vi "Drive Config.vi"(8 "error in (no error)":errorcluster, 11 "Config in":refnum<class "Config.lvclass">) -> (0 "error out":errorcluster, 1 "IDs found?":bool, 2 "Robot Drivetrain Data":T1={"Right"={"Talon"=0, "Victor1"=0, "Victor2"=0}, "Left"={"Talon"=0, "Victor1"=0, "Victor2"=0}, "Drive Velocity Low Gear"={"P"=0.0, "I"=0.0, "D"=0.0, "F"=0.0, "integralZone"=0.0, "allowableClosedLoopError"=0, "maxIntegralAccumulator"=0.0, "closedLoopPeakOutput"=1.0, "closedLoopPeriod"=1}, "Drive Velocity High Gear"={"P"=0.0, "I"=0.0, "D"=0.0, "F"=0.0, "integralZone"=0.0, "allowableClosedLoopError"=0, "maxIntegralAccumulator"=0.0, "closedLoopPeakOutput"=1.0, "closedLoopPeriod"=1}, "Drive Motion Magic Primary Low Gear"={"P"=0.0, "I"=0.0, "D"=0.0, "F"=0.0, "integralZone"=0.0, "allowableClosedLoopError"=0, "maxIntegralAccumulator"=0.0, "closedLoopPeakOutput"=1.0, "closedLoopPeriod"=1}, "Drive Motion Magic Primary High Gear"={"P"=0.0, "I"=0.0, "D"=0.0, "F"=0.0, "integralZone"=0.0, "allowableClosedLoopError"=0, "maxIntegralAccumulator"=0.0, "closedLoopPeakOutput"=1.0, "closedLoopPeriod"=1}, "Drive Motion Magic Secondary Low Gear"={"P"=0.0, "I"=0.0, "D"=0.0, "F"=0.0, "integralZone"=0.0, "allowableClosedLoopError"=0, "maxIntegralAccumulator"=0.0, "closedLoopPeakOutput"=1.0, "closedLoopPeriod"=1}, "Drive Motion Magic Secondary High Gear"={"P"=0.0, "I"=0.0, "D"=0.0, "F"=0.0, "integralZone"=0.0, "allowableClosedLoopError"=0, "maxIntegralAccumulator"=0.0, "closedLoopPeakOutput"=1.0, "closedLoopPeriod"=1}, "Drive Right Invert"=FALSE, "Drive Right Sensor Phase"=FALSE, "Drive Left Invert"=FALSE, "Drive Left Sensor Phase"=FALSE, "Low Gear Max Velocity"=0, "High Gear Max Velocity"=0, "Motion Magic Low Gear Max Velocity"=0, "Motion Magic Low Gear Max Acceleration"=0, "Motion Magic High Gear Max Velocity"=0, "Motion Magic High Gear Max Acceleration"=0}, 3 "Config out":refnum<class "Config.lvclass">, 4 "PIDFs found":bool, 5 "File Found?":bool)   [LabVIEW 2018, in "Config.lvlib" / "Config.lvclass"]
doc: "Use this VI to configure the drive. It will return both if it found the slots, as well as the PIDF values."
uses:
  Config.lvclass
  Controls/Drivetrain Data.ctl
  Drive/Pod Drive/Pod.ctl
  <vilib>/Rock Robotics/WPI/ThirdParty/Phoenix-LabVIEW/Motor Controller/Controls/CTRE_Phoenix_MotorControl_SlotStructure.ctl
  Drive/Pod Drive/Pod Drive.lvclass
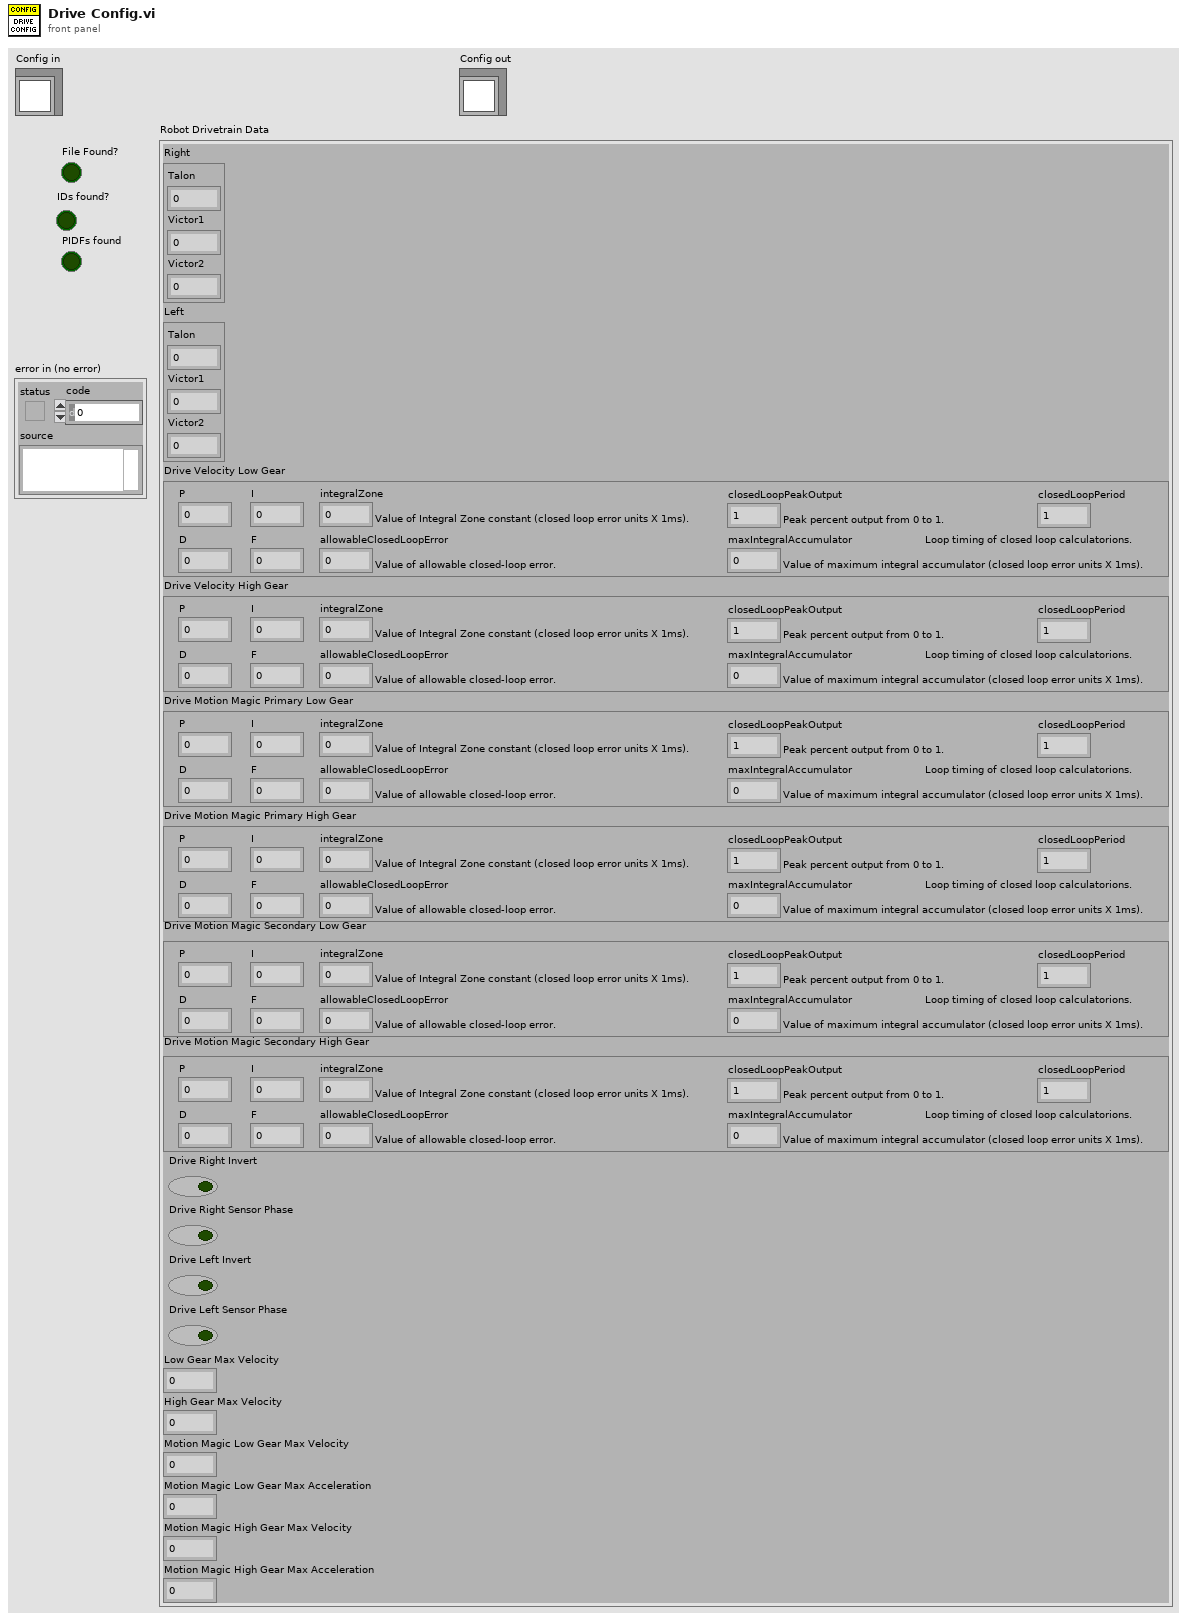
[diagram p1: front panel]
types:
  T1 = typedef "Config.lvlib/Config.lvclass/Drivetrain Data.ctl" = cluster{"Right":T2, "Left":T2, "Drive Velocity Low Gear":T3, "Drive Velocity High Gear":T3, "Drive Motion Magic Primary Low Gear":T3, "Drive Motion Magic Primary High Gear":T3, "Drive Motion Magic Secondary Low Gear":T3, "Drive Motion Magic Secondary High Gear":T3, "Drive Right Invert":bool, "Drive Right Sensor Phase":bool, "Drive Left Invert":bool, "Drive Left Sensor Phase":bool, "Low Gear Max Velocity":u32, "High Gear Max Velocity":u32, "Motion Magic Low Gear Max Velocity":u32, "Motion Magic Low Gear Max Acceleration":u32, "Motion Magic High Gear Max Velocity":u32, "Motion Magic High Gear Max Acceleration":u32}
  T2 = typedef "Drive.lvlib/Pod Drive.lvclass/Pod.ctl" = cluster{"Talon":u8, "Victor1":u8, "Victor2":u8}
  T3 = typedef "CTRE_Phoenix_MotorControl_SlotStructure.ctl" = cluster{"P":dbl, "I":dbl, "D":dbl, "F":dbl, "integralZone":dbl, "allowableClosedLoopError":i32, "maxIntegralAccumulator":dbl, "closedLoopPeakOutput":dbl, "closedLoopPeriod":i32}
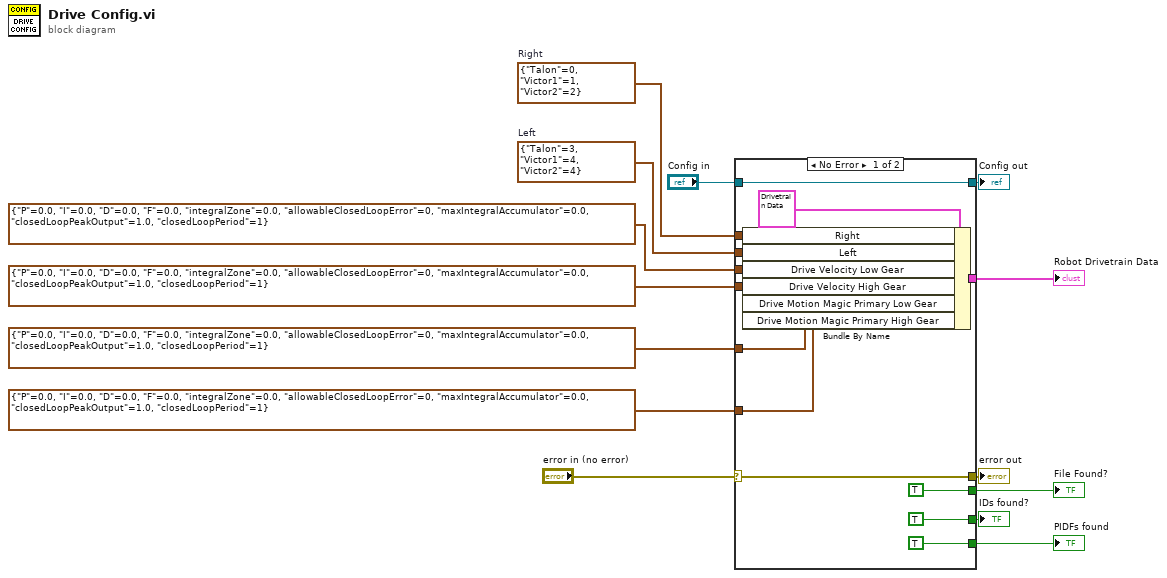
[diagram p0: block diagram]
diagram:
  w1 = T2 {"Talon"=3, "Victor1"=4, "Victor2"=4}  # Left
  w2 = T2 {"Talon"=0, "Victor1"=1, "Victor2"=2}  # Right
  n1 = case shown="No Error" "error in (no error)" {
    selector: "error in (no error)" -> [w26 w29]
    tunnel: [w26 w29] -> w13
    tunnel: [w27 w28] -> w11
    tunnel: "Config in" -> [w27 w28]
    tunnel: [TRUE ("File Found?") _] -> w10
    tunnel: [TRUE ("IDs found?") _] -> w9
    tunnel: [TRUE ("PIDFs found") _] -> w8
    tunnel: [w21 _] -> w7
    tunnel: T3 {"P"=0.0, "I"=0.0, "D"=0.0, "F"=0.0, "integralZone"=0.0, "allowableClosedLoopError"=0, "maxIntegralAccumulator"=0.0, "closedLoopPeakOutput"=1.0, "closedLoopPeriod"=1} ("PID Slot 0") -> [w20 _]
    tunnel: T3 {"P"=0.0, "I"=0.0, "D"=0.0, "F"=0.0, "integralZone"=0.0, "allowableClosedLoopError"=0, "maxIntegralAccumulator"=0.0, "closedLoopPeakOutput"=1.0, "closedLoopPeriod"=1} ("PID Slot 0") -> [w19 _]
    tunnel: T3 {"P"=0.0, "I"=0.0, "D"=0.0, "F"=0.0, "integralZone"=0.0, "allowableClosedLoopError"=0, "maxIntegralAccumulator"=0.0, "closedLoopPeakOutput"=1.0, "closedLoopPeriod"=1} ("PID Slot 0") -> [w18 _]
    tunnel: T3 {"P"=0.0, "I"=0.0, "D"=0.0, "F"=0.0, "integralZone"=0.0, "allowableClosedLoopError"=0, "maxIntegralAccumulator"=0.0, "closedLoopPeakOutput"=1.0, "closedLoopPeriod"=1} ("PID Slot 0") -> [w17 _]
    tunnel: w2 -> [w16 _]
    tunnel: w1 -> [w15 _]
    frame No Error {
      n2 = Bundle By Name(cluster=T1 {"Right"={"Talon"=0, "Victor1"=0, "Victor2"=0}, "Left"={"Talon"=0, "Victor1"=0, "Victor2"=0}, "Drive Velocity Low Gear"={"P"=0.0, "I"=0.0, "D"=0.0, "F"=0.0, "integralZone"=0.0, "allowableClosedLoopError"=0, "maxIntegralAccumulator"=0.0, "closedLoopPeakOutput"=1.0, "closedLoopPeriod"=1}, "Drive Velocity High Gear"={"P"=0.0, "I"=0.0, "D"=0.0, "F"=0.0, "integralZone"=0.0, "allowableClosedLoopError"=0, "maxIntegralAccumulator"=0.0, "closedLoopPeakOutput"=1.0, "closedLoopPeriod"=1}, "Drive Motion Magic Primary Low Gear"={"P"=0.0, "I"=0.0, "D"=0.0, "F"=0.0, "integralZone"=0.0, "allowableClosedLoopError"=0, "maxIntegralAccumulator"=0.0, "closedLoopPeakOutput"=1.0, "closedLoopPeriod"=1}, "Drive Motion Magic Primary High Gear"={"P"=0.0, "I"=0.0, "D"=0.0, "F"=0.0, "integralZone"=0.0, "allowableClosedLoopError"=0, "maxIntegralAccumulator"=0.0, "closedLoopPeakOutput"=1.0, "closedLoopPeriod"=1}, "Drive Motion Magic Secondary Low Gear"={"P"=0.0, "I"=0.0, "D"=0.0, "F"=0.0, "integralZone"=0.0, "allowableClosedLoopError"=0, "maxIntegralAccumulator"=0.0, "closedLoopPeakOutput"=1.0, "closedLoopPeriod"=1}, "Drive Motion Magic Secondary High Gear"={"P"=0.0, "I"=0.0, "D"=0.0, "F"=0.0, "integralZone"=0.0, "allowableClosedLoopError"=0, "maxIntegralAccumulator"=0.0, "closedLoopPeakOutput"=1.0, "closedLoopPeriod"=1}, "Drive Right Invert"=FALSE, "Drive Right Sensor Phase"=FALSE, "Drive Left Invert"=FALSE, "Drive Left Sensor Phase"=FALSE, "Low Gear Max Velocity"=0, "High Gear Max Velocity"=0, "Motion Magic Low Gear Max Velocity"=0, "Motion Magic Low Gear Max Acceleration"=0, "Motion Magic High Gear Max Velocity"=0, "Motion Magic High Gear Max Acceleration"=0} ("Robot Drivetrain Data"), "Right"=w16, "Left"=w15, "Drive Velocity Low Gear"=w20, "Drive Velocity High Gear"=w19, "Drive Motion Magic Primary Low Gear"=w18, "Drive Motion Magic Primary High Gear"=w17) -> (w21:T1)
    }
    frame Error {
    }
  }
  "error out" <- w13
  "Config out" <- w11
  "Robot Drivetrain Data" <- w7
  "File Found?" <- w10
  "IDs found?" <- w9
  "PIDFs found" <- w8
